vi "H5Oget_info_by_idx.vi"(5 "Order":T1 items=["H5_ITER_UNKNOWN"=-1, "H5_ITER_INC"=0, "H5_ITER_DEC"=1], 6 "lapl_id":T7, 7 "Index Field":T2 items=["H5_INDEX_UNKNOWN"=-1, "H5_INDEX_NAME"=0, "H5_INDEX_CRT_ORDER"=1], 8 "error in (no error)":errorcluster, 9 "Index":u64, 10 "Group Name":string=".", 11 "Location Ref":T7) -> (0 "error out":errorcluster, 2 "H5O_info_t":T3 {"H5O_hdr_info_t"."mesg"."shared" format="%.0x"; "H5O_hdr_info_t"."mesg"."present" format="%.0x"; "H5O_hdr_info_t"."flags" format="%.0x"; "type" items=["H5O_TYPE_UNKNOWN"=-1, "H5O_TYPE_GROUP"=0, "H5O_TYPE_DATASET"=1, "H5O_TYPE_NAMED_DATATYPE"=2]}, 3 "Location Ref out":T7)   [LabVIEW 2017]
doc: "Retrieves the metadata for an object, \n identifying the object by an index position."
uses:
  <vilib>/UPVI/lvhdf5/library.llb/HDF5 Ref.ctl
  <vilib>/UPVI/lvhdf5/object.llb/LVH5O_info_t.ctl
  <vilib>/UPVI/lvhdf5/object.llb/H5O_type_t.ctl
  <vilib>/UPVI/lvhdf5/object.llb/H5O_hdr_info_t.ctl
  <vilib>/UPVI/lvhdf5/library.llb/H5_ih_info_t.ctl
  <vilib>/UPVI/lvhdf5/library.llb/H5_index_t.ctl
  <vilib>/UPVI/lvhdf5/library.llb/H5_iter_order_t.ctl
  <vilib>/UPVI/lvhdf5/object.llb/H5O_info_t.ctl
  <vilib>/UPVI/lvhdf5/hdf5.dll
panel:
  # "LVHDF5 Toolkit\nCopyright (c) 2005-2013 by Jason D. Sommerville\nCopyright (c) 2014-2015 by UPVI, LLC.\n\nThis use and distribution of this file is governed by the terms found in \nLICENSE.txt distributed with this toolkit and installed at\n <user.lib>\\_lvhdf5\\LICENSE.txt"
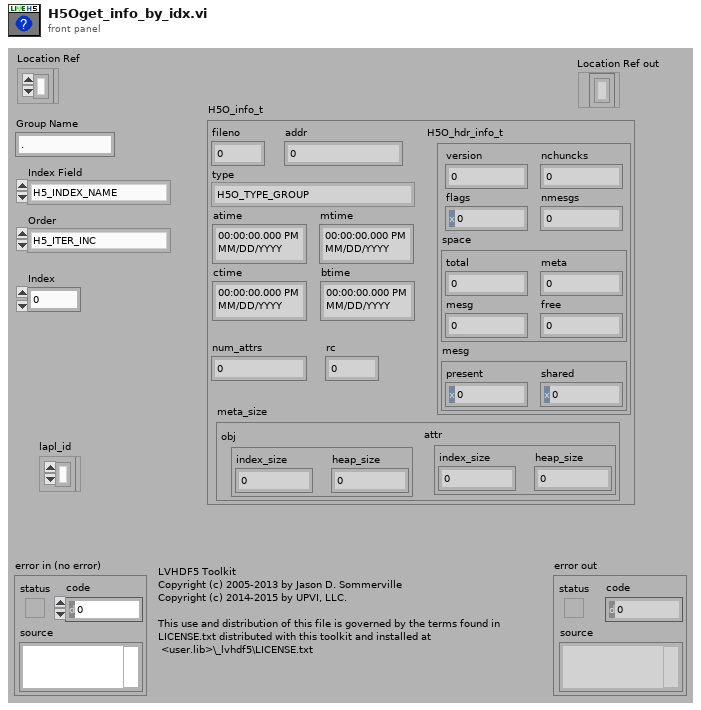
[diagram p1: front panel]
types:
  T1 = typedef "H5_iter_order_t.ctl" = i32
  T2 = typedef "H5_index_t.ctl" = i32
  T3 = typedef "LVH5O_info_t.ctl" = cluster{"fileno":u32, "addr":u64, "type":T4, "rc":u32, "atime":timestamp, "mtime":timestamp, "ctime":timestamp, "btime":timestamp, "num_attrs":i64, "H5O_hdr_info_t":T5, "meta_size":cluster{"obj":T6, "attr":T6}}
  T4 = typedef "H5O_type_t.ctl" = i32
  T5 = typedef "H5O_hdr_info_t.ctl" = cluster{"version":u32, "nmesgs":u32, "nchuncks":u32, "flags":u32, "space":cluster{"total":u64, "meta":u64, "mesg":u64, "free":u64}, "mesg":cluster{"present":u64, "shared":u64}}
  T6 = typedef "H5_ih_info_t.ctl" = cluster{"index_size":u64, "heap_size":u64}
  T7 = typedef "HDF5 Ref.ctl" = refnum<k1>
  T8 = typedef "H5O_info_t.ctl" = cluster{"fileno":u32, "unused":u32, "addr":u64, "type":T4, "rc":u32, "atime":i64, "mtime":i64, "ctime":i64, "btime":i64, "num_attrs":i64, "H5O_hdr_info_t":T5, "meta_size":cluster{"obj":T6, "attr":T6}}
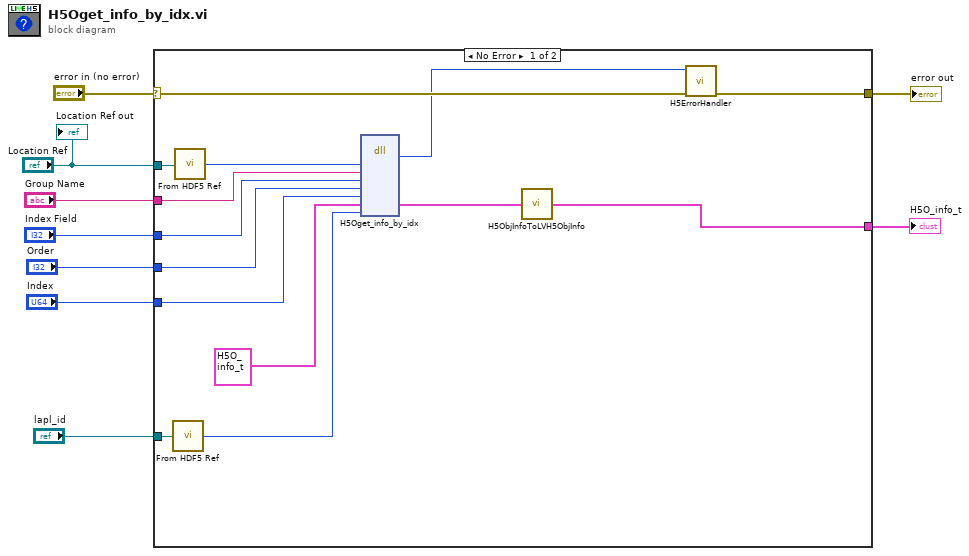
[diagram p0: block diagram]
diagram:
  n1 = case shown="No Error" "error in (no error)" {
    selector: "error in (no error)" -> [w23 w24]
    tunnel: [w22 w24] -> w8
    tunnel: "lapl_id" -> [w21 _]
    tunnel: "Location Ref" -> [w18 _]
    tunnel: "Group Name" -> [w16 _]
    tunnel: [w10 _] -> w4
    tunnel: "Index Field" -> [w15 _]
    tunnel: "Order" -> [w14 _]
    tunnel: "Index" -> [w13 _]
    frame No Error {
      n2 = call <vilib>:"From HDF5 Ref.vi"("HDF5 Ref"=w21) -> ("I32"=w20:i32)
      n3 = call <vilib>:"From HDF5 Ref.vi"("HDF5 Ref"=w18) -> ("I32"=w17:i32)
      n4 = dll-call lib="C:/Program Files/National Instruments/LabVIEW 2017/vi.lib/UPVI/lvhdf5/hdf5.dll" fn="H5Oget_info_by_idx"("loc_id"=w17, "group_name"=w16, "index_field"=w15, "order"=w14, "n"=w13, "link_buff"=T8 {"fileno"=0, "unused"=0, "addr"=0, "type"=0, "rc"=0, "atime"=0, "mtime"=0, "ctime"=0, "btime"=0, "num_attrs"=0, "H5O_hdr_info_t"={"version"=0, "nmesgs"=0, "nchuncks"=0, "flags"=0, "space"={"total"=0, "meta"=0, "mesg"=0, "free"=0}, "mesg"={"present"=0, "shared"=0}}, "meta_size"={"obj"={"index_size"=0, "heap_size"=0}, "attr"={"index_size"=0, "heap_size"=0}}} ("info"), "lapl_id"=w20) -> ("return type"=w19:i32, "link_buff"=w11:T8)  [unwired: 9 in, 2 out]
      n5 = call <vilib>:"H5ObjInfoToLVH5ObjInfo.vi"("H5O_info_t"=w11) -> ("LVH5O_info_t"=w10:T3)
      n6 = call <vilib>:"H5ErrorHandler.vi"("error in (no error)"=w23, "herr_t"=w19) -> ("error out"=w22:errorcluster)  [unwired: 3 in, 4 out]
    }
    frame Error {
    }
  }
  "error out" <- w8
  "H5O_info_t" <- w4
  "Location Ref out" <- "Location Ref"
